vi "_DServerDevicePropertyToDoubleArray.vi"(3 "error in":errorcluster, 4 "property name":string, 5 "device name":string) -> (0 "error out":errorcluster, 1 "property value":dbl[](array[numeric]))   [LabVIEW 2014, in "tango.lvlib"]
uses:
  tango.lvlib
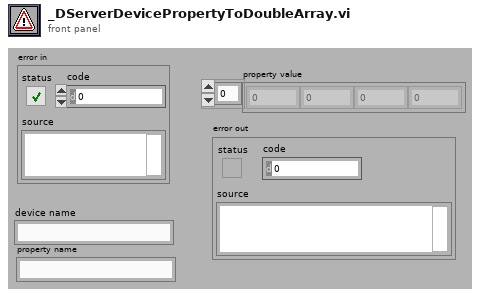
[diagram p1: front panel]
types:
  T1 = typedef "tango.lvlib/_DeviceProperty.ctl" = cluster{"Name":string, "Data":u8[], "Tango Data Type":T2}
  T2 = typedef "tango.lvlib/_DataType.ctl" = enum16{"STATE_SCA", "STATE_SPE", "STATE_IMG", "STRING_SCA", "STRING_SPE", "STRING_IMG", "BOOL_SCA", "BOOL_SPE", "BOOL_IMG", "UCHAR_SCA", "UCHAR_SPE", "UCHAR_IMG", "SHORT_SCA", "SHORT_SPE", "SHORT_IMG", "USHORT_SCA", "USHORT_SPE", "USHORT_IMG", "LONG_SCA", "LONG_SPE", "LONG_IMG", "ULONG_SCA", "ULONG_SPE", "ULONG_IMG", "LONG64_SCA", "LONG64_SPE", "LONG64_IMG", "ULONG64_SCA", "ULONG64_SPE", "ULONG64_IMG", "FLOAT_SCA", "FLOAT_SPE", "FLOAT_IMG", "DOUBLE_SCA", "DOUBLE_SPE", "DOUBLE_IMG", "SCA_ENCODED", "SPE_ENCODED", "IMG_ENCODED", "UNKNOWN_DATA_TYPE"}
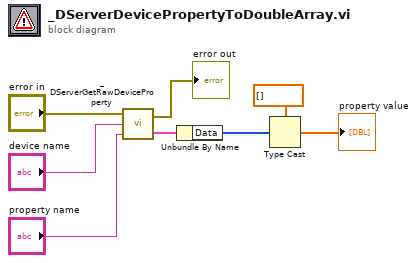
[diagram p0: block diagram]
diagram:
  n1 = call "_DServerGetRawDeviceProperty.vi"("property_name"="property name", "device_name"="device name", "error in"="error in") -> ("property_value"=w5:T1, "error out"=→"error out":errorcluster)
  n2 = Unbundle By Name(w5) -> ("Data"=w2:u8[])
  n3 = Type Cast(type=dbl[] [], x=w2) -> (*(type *) &x=→"property value":dbl[])
